vi "Intake Testt.vi"   [LabVIEW 2018]
uses:
  Floating Intake/Implementation/Floating Intake Operations.ctl
  <vilib>/Rock Robotics/Network Tables/NT Write String.vi
types:
  T1 = typedef "Floating Intake Operations.ctl" = enum16{"Reserve", "Read Current", "Immediate", "Duration"}
  T2 = typedef "Command Status Info.ctl" = cluster{"Name":string, "Status":T3, "notifier out":T4}
  T3 = typedef "Completion Status.ctl" = enum16{"Successful", "Aborted", "Incomplete"}
  T4 = typedef "Completion Notifier.ctl" = refnum<notifier>
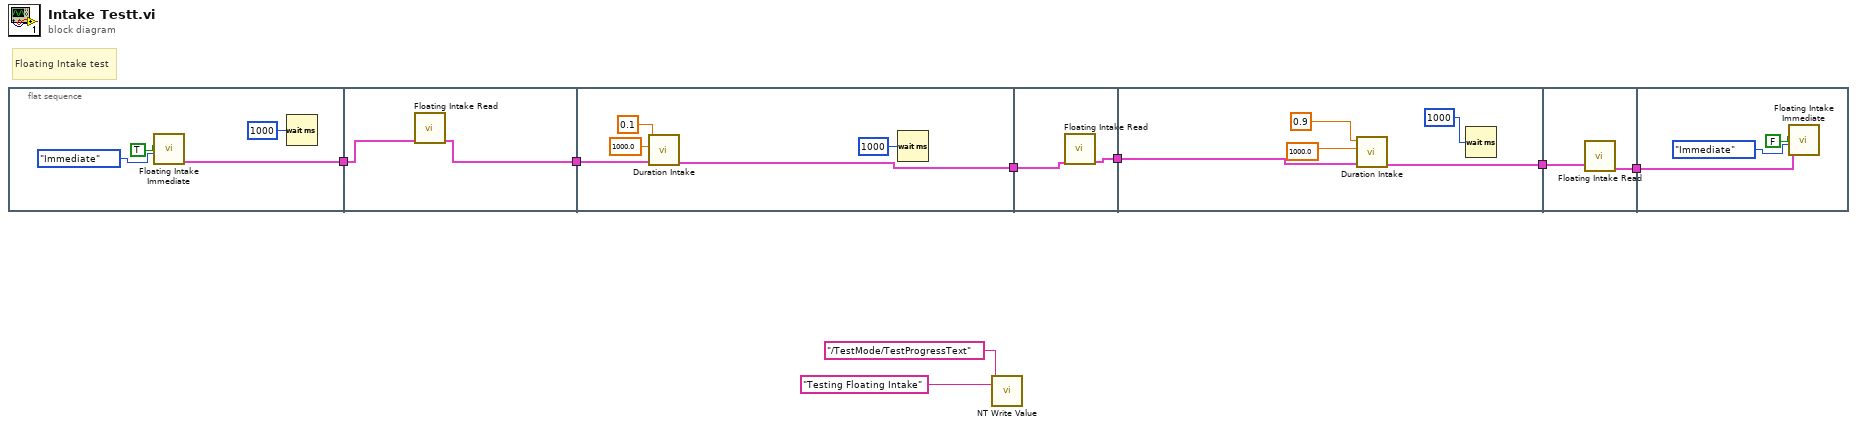
[diagram p0: block diagram]
diagram:
  # "Floating Intake test"
  n1 = flat-sequence {
    tunnel: [w10] -> w8
    tunnel: w8 -> [w14]
    tunnel: [w13] -> w7
    tunnel: w7 -> [w19]
    tunnel: [w15] -> w6
    tunnel: w6 -> [w21]
    tunnel: [w20] -> w5
    tunnel: w5 -> [w24]
    tunnel: [w23] -> w4
    tunnel: w4 -> [w28]
    tunnel: [w27] -> w3
    tunnel: w3 -> [w29]
    frame #0 {
      n2 = call "Floating Intake Immediate.vi"("Operation"=Floating_Intake_Operations."Immediate", "extend"=TRUE) -> ("Command Info Out"=w10:T2)  [unwired: 9 in]
      n3 = Wait (ms)(milliseconds to wait=u32 1000) -> ()  [unwired: 1 out]
    }
    frame #1 {
      n4 = call "Floating Intake Read.vi"("Command Info In"=w14) -> ("Command Info Out"=w13:T2)  [unwired: 9 in, 1 out]
    }
    frame #2 {
      n5 = call "Duration Intake.vi"("Command Info In"=w19, "Duration (s)"=1000.0, "Setpoint"=0.1) -> ("Command Info Out"=w15:T2)  [unwired: 8 in]
      n6 = Wait (ms)(milliseconds to wait=u32 1000) -> ()  [unwired: 1 out]
    }
    frame #3 {
      n7 = call "Floating Intake Read.vi"("Command Info In"=w21) -> ("Command Info Out"=w20:T2)  [unwired: 9 in, 1 out]
    }
    frame #4 {
      n8 = call "Duration Intake.vi"("Command Info In"=w24, "Duration (s)"=1000.0, "Setpoint"=0.9) -> ("Command Info Out"=w23:T2)  [unwired: 8 in]
      n9 = Wait (ms)(milliseconds to wait=u32 1000) -> ()  [unwired: 1 out]
    }
    frame #5 {
      n10 = call "Floating Intake Read.vi"("Command Info In"=w28) -> ("Command Info Out"=w27:T2)  [unwired: 9 in, 1 out]
    }
    frame #6 {
      n11 = call "Floating Intake Immediate.vi"("Command Info In"=w29, "Operation"=Floating_Intake_Operations."Immediate", "extend"=FALSE) -> ()  [unwired: 8 in, 1 out]
    }
  }
  n12 = call-poly <vilib>:"NT Write Value.vi"("String"="Testing Floating Intake", "Name"="/TestMode/TestProgressText") -> ()  [unwired: 9 in, 1 out]
